vi "Test Coffee Shop Remove Cashier Broadcast Name.vi"(8 "error in (no error)":errorcluster, 11 "Coffee Shop Test In":refnum<class "Coffee Shop Test.lvclass">=refnum) -> (0 "error out":errorcluster, 3 "Coffee Shop Test Out":refnum<class "Coffee Shop Test.lvclass">)   [LabVIEW 2020, in "Coffee Shop Test.lvclass"]
uses:
  Coffee Shop Test.lvclass
  Processes/Coffee Shop/Coffee Shop.lvclass
  <vilib>/Astemes/Triarc Framework/Process/Process.lvclass
  C:/Program Files (x86)/National Instruments/LabVIEW 2020/vi.lib/Astemes/Triarc Framework/Application/Application.lvclass
  C:/Program Files (x86)/National Instruments/LabVIEW 2020/vi.lib/Astemes/Triarc Framework/Process/Process.lvclass
  C:/Program Files (x86)/National Instruments/LabVIEW 2020/vi.lib/Astemes/Triarc Framework/Base/Base.lvclass
  C:/Program Files (x86)/National Instruments/LabVIEW 2020/vi.lib/Astemes/Triarc Framework/Error Handler Interface/Error Handler Interface.lvclass
  C:/Program Files (x86)/National Instruments/LabVIEW 2020/vi.lib/Astemes/Triarc Framework/Logging/Logging.lvclass
  C:/Program Files (x86)/National Instruments/LabVIEW 2020/vi.lib/Astemes/Triarc Framework/Async Handler/Async Handler.lvclass
  C:/git/astemes-triarc-examples/source/Coffee Shop/Processes/Coffee Shop/Coffee Shop.lvclass
  8d2e8d5f-5d0f-4752-985f-4bfcb05e8165.vi
  <vilib>/Astemes/Triarc Framework/Support/Broadcast Event Dequeuers.lvlib
  <vilib>/Astemes/LUnit/Test Case.lvclass
  C:/Program Files (x86)/National Instruments/LabVIEW 2020/vi.lib/Astemes/LUnit/Test Case.lvclass
  C:/Program Files (x86)/National Instruments/LabVIEW 2020/vi.lib/Astemes/LUnit/LUnit Runnable.lvclass
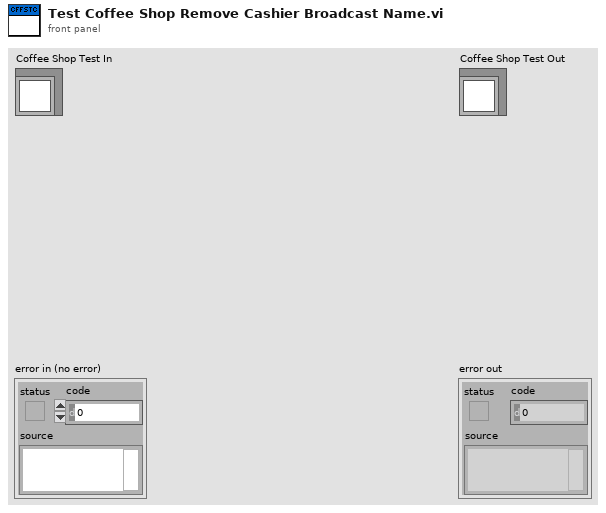
[diagram p1: front panel]
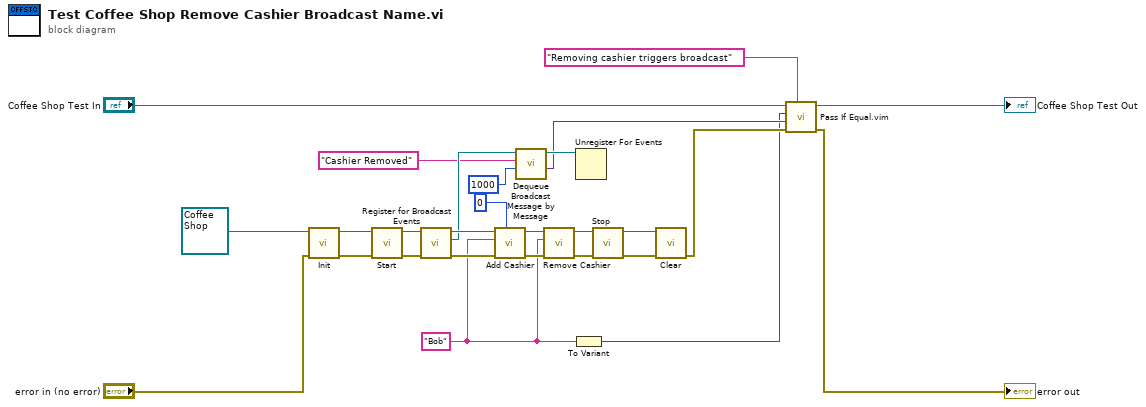
[diagram p0: block diagram]
diagram:
  w2 = "Bob" ("Name")
  n1 = call-dynamic "Init.vi"("error in (no error)"="error in (no error)", "Process In"=refnum<class "Coffee Shop.lvclass"> refnum ("Coffee Shop.lvclass")) -> ("error out"=w25:errorcluster, "Process Out"=w26:refnum<class "Coffee Shop.lvclass">)  [unwired: 8 in]
  n2 = call <vilib>:"Start.vi"("error in (no error)"=w25, "Process In"=w26) -> ("error out"=w24:errorcluster, "Process Out"=w18:refnum<class "Coffee Shop.lvclass">)  [unwired: 7 in, 1 out]
  n3 = call <vilib>:"Register for Broadcast Events.vi"("error in (no error)"=w24, "Process In"=w18) -> ("error out"=w19:errorcluster, "Event Registration Refnum Out"=w16:refnum<event-registration>, "Process Out"=w17:refnum<class "Coffee Shop.lvclass">)  [unwired: 7 in]
  n4 = call "Add Cashier.vi"("Time Scale [ms]"=u32 0, "error in (no error)"=w19, "Name"=w2, "Coffee Shop in"=w17) -> ("error out"=w20:errorcluster, "Coffee Shop out"=w4:refnum<class "Coffee Shop.lvclass">)  [unwired: 6 in]
  n5 = call <vilib>:"Dequeue Broadcast Message by Message.vi"("Timeout (-1)"=1000, "Message"="Cashier Removed", "Event Registration Refnum"=w16) -> ("Message Data"=w7:variant, "Event Registration Refnum Out"=w14:refnum<event-registration>)  [unwired: 4 in, 3 out]
  n6 = call "Remove Cashier.vi"("error in (no error)"=w20, "Name"=w2, "Coffee Shop In"=w4) -> ("error out"=w5:errorcluster, "Coffee Shop Out"=w3:refnum<class "Coffee Shop.lvclass">)  [unwired: 7 in]
  n7 = To Variant(anything=w2) -> (Variant=w6:variant)
  n8 = Unregister For Events(event registration refnum=w14) -> ()  [unwired: 1 in, 1 out]
  n9 = call <vilib>:"Stop.vi"("error in (no error)"=w5, "Process In"=w3) -> ("error out"=w22:errorcluster, "Process Out"=w23:refnum<class "Coffee Shop.lvclass">)  [unwired: 7 in, 1 out]
  n10 = call-dynamic "Clear.vi"("error in (no error)"=w22, "Application In"=w23) -> ("error out"=w10:errorcluster)  [unwired: 9 in]
  n11 = call "Pass If Equal.vim"("Description"="Removing cashier triggers broadcast", "error in (no error)"=w10, "Actual"=w7, "Expected"=w6, "LUnit Test Case In"="Coffee Shop Test In") -> ("error out"=→"error out":errorcluster, "LUnit Test Case Out"=→"Coffee Shop Test Out":refnum<class "Test Case.lvclass">)  [unwired: 5 in]
